vi "get remaining time budget.vi"(8 "error in":errorcluster, 10 "dt":u32=1, 11 "timing source in":refnum<class "DAQmx Single Point HW Timed.lvclass">) -> (0 "error out":errorcluster, 2 "budget (ns)":u64, 3 "timing source out":refnum<class "DAQmx Single Point HW Timed.lvclass">)   [LabVIEW 2014, in "DAQmx Single Point HW Timed.lvclass"]
uses:
  DAQmx Single Point HW Timed.lvclass
  <vilib>/NI/Module Timing Source/timing source/TBM timing source.lvclass
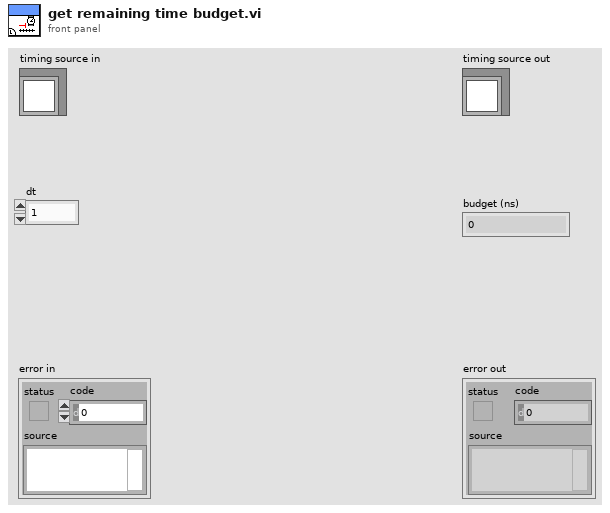
[diagram p1: front panel]
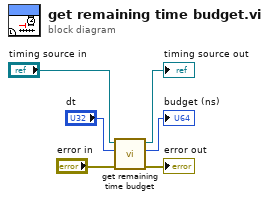
[diagram p0: block diagram]
diagram:
  n1 = call-parent "get remaining time budget.vi"("error in"="error in", "dt"="dt", "timing source in"="timing source in") -> ("error out"=→"error out":errorcluster, "budget (ns)"=→"budget (ns)":u64, "timing source out"=→"timing source out":refnum<class "DAQmx Single Point HW Timed.lvclass">)  [unwired: 6 in]
